vi "_indexArray.vi"(7 "xData":dbl[](array[numeric]), 11 "index":i32) -> (3 "Data Point":dbl)   [LabVIEW 2015]
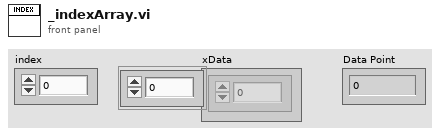
[diagram p1: front panel]
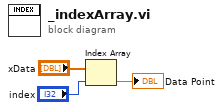
[diagram p0: block diagram]
diagram:
  n1 = Index Array(array="xData", index="index") -> (element=→"Data Point":dbl)
